vi "edge_to_node_ids.vi"(10 "edge":refnum<class "Edge.lvclass">) -> (2 "node-ids-cluster":T1)   [LabVIEW 2020, in "graph.lvlib" / "Graph.lvclass"]
uses:
  Graph.lvclass
  edge-definition-cluster.ctl
  ID/ID.lvclass
  Edge/Edge.lvclass
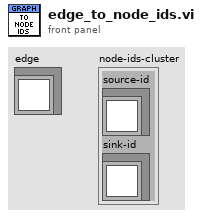
[diagram p1: front panel]
types:
  T1 = typedef "graph.lvlib/Graph.lvclass/edge-definition-cluster.ctl" = cluster{"source-id":refnum<class "ID.lvclass">, "sink-id":refnum<class "ID.lvclass">}
  T2 = cluster{"source-id":refnum<class "ID.lvclass">, "sink-id":refnum<class "ID.lvclass">}
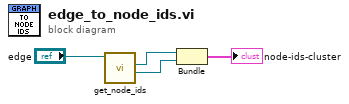
[diagram p0: block diagram]
diagram:
  n1 = call "get_node_ids.vi"("edge"="edge") -> ("sink-id"=w3:refnum<class "ID.lvclass">, "source-id"=w2:refnum<class "ID.lvclass">)  [unwired: 9 in]
  n2 = Bundle("source-id"=w2, "sink-id"=w3) -> (→"node-ids-cluster":T2)  [unwired: 1 in]
